vi "update config.vi"(8 "error in (no error)":errorcluster, 10 "user configurations":T1={"vst_device"=["VST_1", "VST_2"], "RF gain "=10.0, "buffer size"=524288, "center frequency (Hz) "=1000000000.0, "P2P sample rate"=200000000.0, "mode"=enum."5785 - 2*180MHz", "devicess"=["IF_transiver_0", "IF_transiver_1", "IF_transiver_2"], "gen for df"=FALSE, "Rx settings"={"min PW         "=0.0, "max gap        "=0.0, "detection bar"=0.0, "peak detect                        "=FALSE}}, 11 "pulse_gen_and_detect_p2p in":refnum<class "pulse_gen_and_detect_p2p.lvclass">) -> (0 "error out":errorcluster, 1 "min frequency":dbl, 2 "max frequency":dbl, 3 "pulse_gen_and_detect_p2p out":refnum<class "pulse_gen_and_detect_p2p.lvclass">)   [LabVIEW 2021, in "pulse_gen_and_detect_p2p.lvclass"]
uses:
  pulse_gen_and_detect_p2p.lvclass
  pulse_tx_vis/CTL/user config.ctl
  <vilib>/userdefined/High Color/nirio_resource_hc.ctl
  pulse_gen_and_detect_p2p.lvclass/pulse_gen_and_detect_p2p.ctl
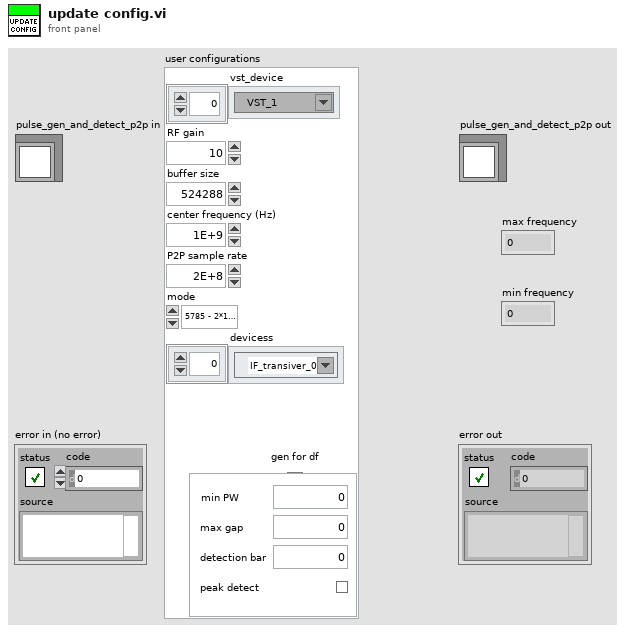
[diagram p1: front panel]
types:
  T1 = typedef "user config.ctl" = cluster{"vst_device":refnum<k15>[], "RF gain ":dbl, "buffer size":u32, "center frequency (Hz) ":dbl, "P2P sample rate":dbl, "mode":enum16{"USRP - 180MHz", "5785 - 2*180MHz", "5785 - 3.2GHz", "P2P - VST"}, "devicess":T2[], "gen for df":bool, "Rx settings":cluster{"min PW         ":dbl, "max gap        ":dbl, "detection bar":dbl, "peak detect                        ":bool}}
  T2 = typedef "nirio_resource_hc.ctl" = tag
  T3 = cluster{"min PW (fft cycels)":u16, "max PW (fft cycels)":u16, "max gap (fft cycels)":u8, "detection bar (liniar amp)":fxp<+,64,63>, "peak detect":bool}
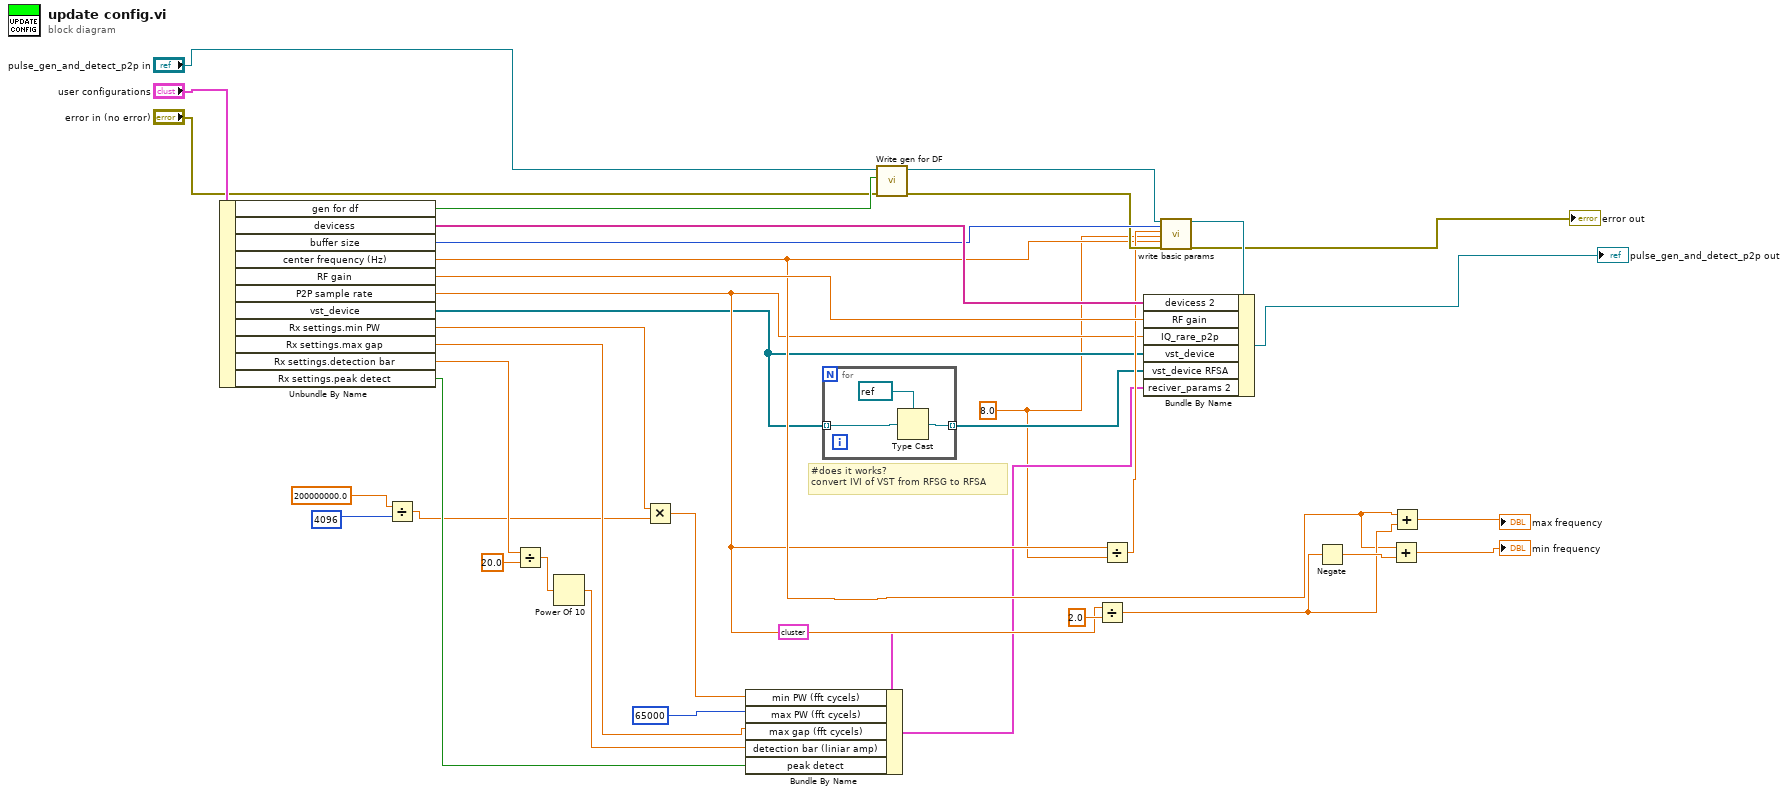
[diagram p0: block diagram]
diagram:
  w13 = 8.0 ("t")
  # "#does it works?\nconvert IVI of VST from RFSG to RFSA"
  n1 = Unbundle By Name("user configurations") -> ("gen for df"=w33:bool, "devicess"=w37:T2[], "buffer size"=w36:u32, "center frequency (Hz)"=w26:dbl, "RF gain"=w31:dbl, "P2P sample rate"=w25:dbl, "vst_device"=w17:refnum<k15>[], "Rx settings.min PW"=w3:dbl, "Rx settings.max gap"=w7:dbl, "Rx settings.detection bar"=w10:dbl, "Rx settings.peak detect"=w12:bool)
  n2 = Divide(x=200000000.0 ("y"), y=4096) -> (x/y=w2:dbl)
  n3 = Divide(x=w10, y=20.0) -> (x/y=w9:dbl)
  n4 = Power Of 10(x=w9) -> (10^x=w8:dbl)
  n5 = Multiply(x=w3, y=w2) -> (x*y=w1:dbl)
  n6 = Bundle By Name(cluster=T3 {"min PW (fft cycels)"=0, "max PW (fft cycels)"=0, "max gap (fft cycels)"=0, "detection bar (liniar amp)"=0.0, "peak detect"=FALSE} ("reciver_params 2"), "min PW (fft cycels)"=w1, "max PW (fft cycels)"=u16 65000, "max gap (fft cycels)"=w7, "detection bar (liniar amp)"=w8, "peak detect"=w12) -> (w14:T3)
  n7 = for {
    tunnel: w17 -> [w40] mode=indexing
    tunnel: [w39] -> w16 mode=indexing
    n8 = Type Cast(type=refnum<k15> refnum ("resource name"), x=w40) -> (*(type *) &x=w39:refnum<k15>)
  }
  n9 = call-dynamic "Write gen for DF.vi"("error in (no error)"="error in (no error)", "gen for DF"=w33, "device_type in"="pulse_gen_and_detect_p2p in") -> ("error out"=w32:errorcluster, "device_type out"=w34:refnum<class "pulse_gen_and_detect_p2p.lvclass">)  [unwired: 7 in]
  n10 = Divide(x=w25, y=2.0) -> (x/y=w29:dbl)
  n11 = Divide(x=w25, y=w13) -> (x/y=w27:dbl)
  n12 = call-dynamic "write basic params.vi"("device_type in"=w34, "buffer size"=w36, "Fs  FPGA"=w27, "SPC"=w13, "center frequency (Hz)"=w26, "error in (no error)"=w32) -> ("device_type out"=w35:refnum<class "pulse_gen_and_detect_p2p.lvclass">, "error out"=→"error out":errorcluster)  [unwired: 12 in]
  n13 = Bundle By Name(cluster=w35, "devicess 2"=w37, "RF gain"=w31, "IQ_rare_p2p"=w25, "vst_device"=w17, "vst_device RFSA"=w16, "reciver_params 2"=w14) -> (→"pulse_gen_and_detect_p2p out":refnum<class "pulse_gen_and_detect_p2p.lvclass">)
  n14 = Negate(x=w29) -> (-x=w30:dbl)
  n15 = Add(x=w26, y=w30) -> (x+y=→"min frequency":dbl)
  n16 = Add(x=w26, y=w29) -> (x+y=→"max frequency":dbl)
